vi "Host__MainNewS.vi"() -> ()   [LabVIEW 2018]
uses:
  Master/DAQ/Master_DataControl.ctl
  Master/DAQ/TypeDef_cRIOData.ctl
  Master/IMU/TypeDef_IMUData.ctl
  Master/CAN/TypeDef_BMSData.ctl
  Master/CAN/TypeDef_BMS_Status.ctl
  Master/CAN/MotorController/fixedMotorData.ctl
  Master/CAN/MotorController/MotorStatus.ctl
  Master/Control/TypeDef_DigitalOuts.ctl
  Libraries/TypeDef_CurrentState.ctl
  HealthCheckClass/HealthCheck.lvclass
panel:
  out "Low Side Indicator":bool
  out "Precharge Indicator":bool
  out "Dump Valve":bool
  out "Ignition Indicator":bool
  out "Pump Indicator":bool
  out "High Side Indicator":bool
  out "Clamp Indicator":bool
  out "Brakes Indicator":bool
  out "Pod Power":bool
  out "x Acceleration (g)":dbl(graph)
  out "Speed (mph)":dbl(graph)
  in  "ManualBrake":bool
  in  "ForceIdle":bool
  in  "Pod Power":bool
  out "CurrentState Ind.":u16(ring)
  in  "stop":bool
  in  "Edit Table":bool
  out "HealthCheckTable":string[][](table)
  in  "Tab Control":enum32{"Service", "Systems Check", "Run"}(tab)
  in  "DrvieEnable":bool
  in  "ServiceHOLD":bool
  in  "Service Toggle":bool
  in  "Ignition":bool
  in  "HighSidePermission (SC)":bool caption="High\nSide"
  in  "Brakes (SC)":bool
  in  "Clamp (SC)":bool
  in  "Pump (SC)":bool
  in  "Ignition (SC)":bool
  in  "Low Side (SC)":bool
  in  "Pre-Charge (SC)":bool
  in  "High Side (SC)":bool
  in  "DriveEnable(SC)":bool
  in  "Motor Controller":bool
  in  "Pre-charge":bool
  in  "Ready":bool
  in  "Launch":bool
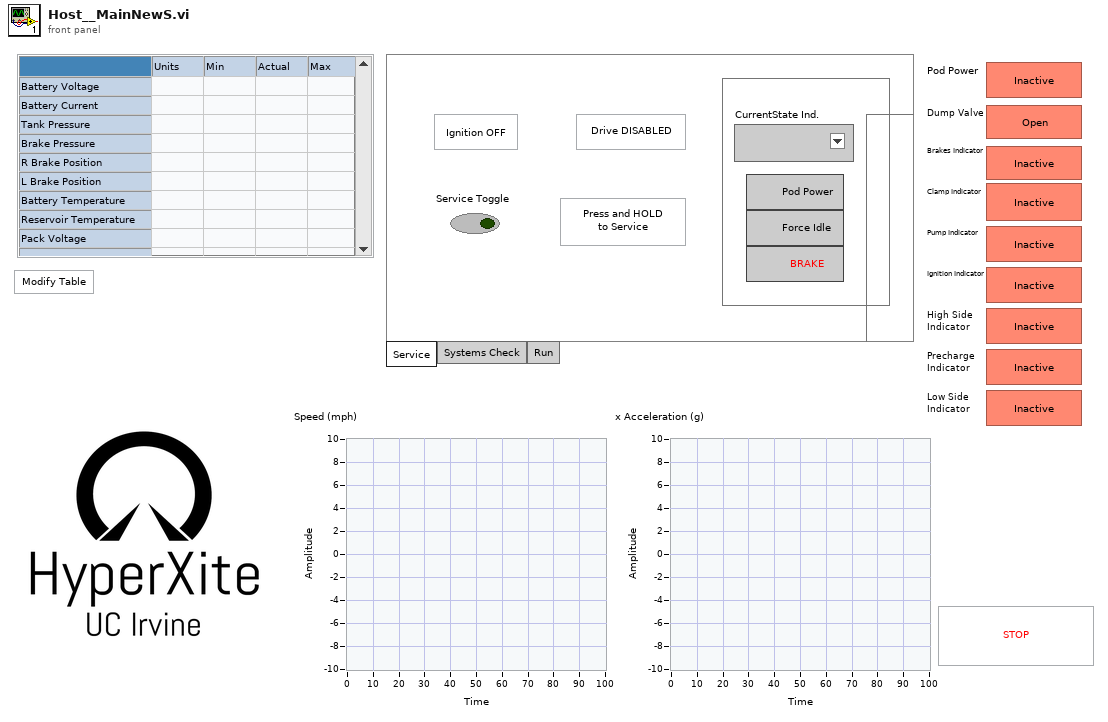
[diagram p1: front panel]
types:
  T1 = enum8{"Enabled", "Disabled", "Disabled and Grayed Out"}
  T2 = typedef "TypeDef_DigitalOuts.ctl" = cluster{"Pod Power":bool, "Dump Valve":bool, "Brakes":bool, "Clamp":bool, "Pump":bool, "Ignition":bool, "DO6":bool, "DO7":bool, "HighSide":bool, "Precharge":bool, "LowSide":bool, "DO3":bool, "DO4":bool, "DO5":bool, "DO62":bool, "DO72":bool}
  T3 = typedef "Master_DataControl.ctl" = cluster{"cRIO Data":T4, "IMU Data":T5, "BMS Data":T6, "Motor Data":T8}
  T4 = typedef "TypeDef_cRIOData.ctl" = cluster{"Time (ms)":dbl, "24V Battery (V)":dbl, "LowV Current (A)":dbl, "Fiducial Sensor (V)":dbl, "PV Pressure (psig)":dbl, "Flow Sensor (V)":dbl, "Temp Fairing (F)":dbl, "Temp Reservoir (F)":dbl, "HallEffect Right (in)":dbl, "HallEffect Left (in)":dbl, "PT Tank (psig)":dbl, "PT Clamp Right (psig)":dbl, "PT Clamp Left (psig)":dbl, "PT Brake (psig)":dbl, "PT Cooling (psig)":dbl, "Displacement (ft)":dbl, "Velocity (ft/s)":dbl}
  T5 = typedef "TypeDef_IMUData.ctl" = cluster{"x acceleration (g)":dbl, "Pressure (psia)":dbl, "Temperature (F)":dbl}
  T6 = typedef "TypeDef_BMSData.ctl" = cluster{"Max Cell Voltage (V)":dbl, "Max Cell ID":dbl, "Min Cell Voltage (V)":dbl, "Min Cell ID":dbl, "State of Charge (%)":dbl, "Average Voltage (V)":dbl, "Voltage Delta (V)":dbl, "Pack Current (A)":dbl, "Pack Voltage (V)":dbl, "Max Resistance (Ohm)":dbl, "Min Resistance (Ohm)":dbl, "Average Resistance (Ohm)":dbl, "Delta Resistance (Ohm)":dbl, "Highest Temperature(F)":dbl, "BmsStatus":T7}
  T7 = typedef "TypeDef_BMS_Status.ctl" = cluster{"isFault":bool, "isolationMonitoring":bool}
  T8 = typedef "fixedMotorData.ctl" = cluster{"Velo (RPM)":dbl, "MotorTemp(F)":dbl, "CtrlTemp(F)":dbl, "DcLinkVolt(V)":dbl, "ErrorCode":dbl, "motorStatus":T9, "isAlive":bool, "motorControllerState":u16}
  T9 = typedef "MotorStatus.ctl" = cluster{"isReady":bool, "isOn":bool, "isOperEn":bool, "isFault":bool, "isVoltEn":bool, "targetReached":bool, "isWarning":bool}
  T10 = typedef "TypeDef_CurrentState.ctl" = enum16{"Fault", "Idle", "Ready", "Pushing", "Coast", "Braking"}
  T11 = typedef "HealthCheck.lvclass/HCState_TypeDef.ctl" = enum16{"Initialization", "Running", "Modify Table"}
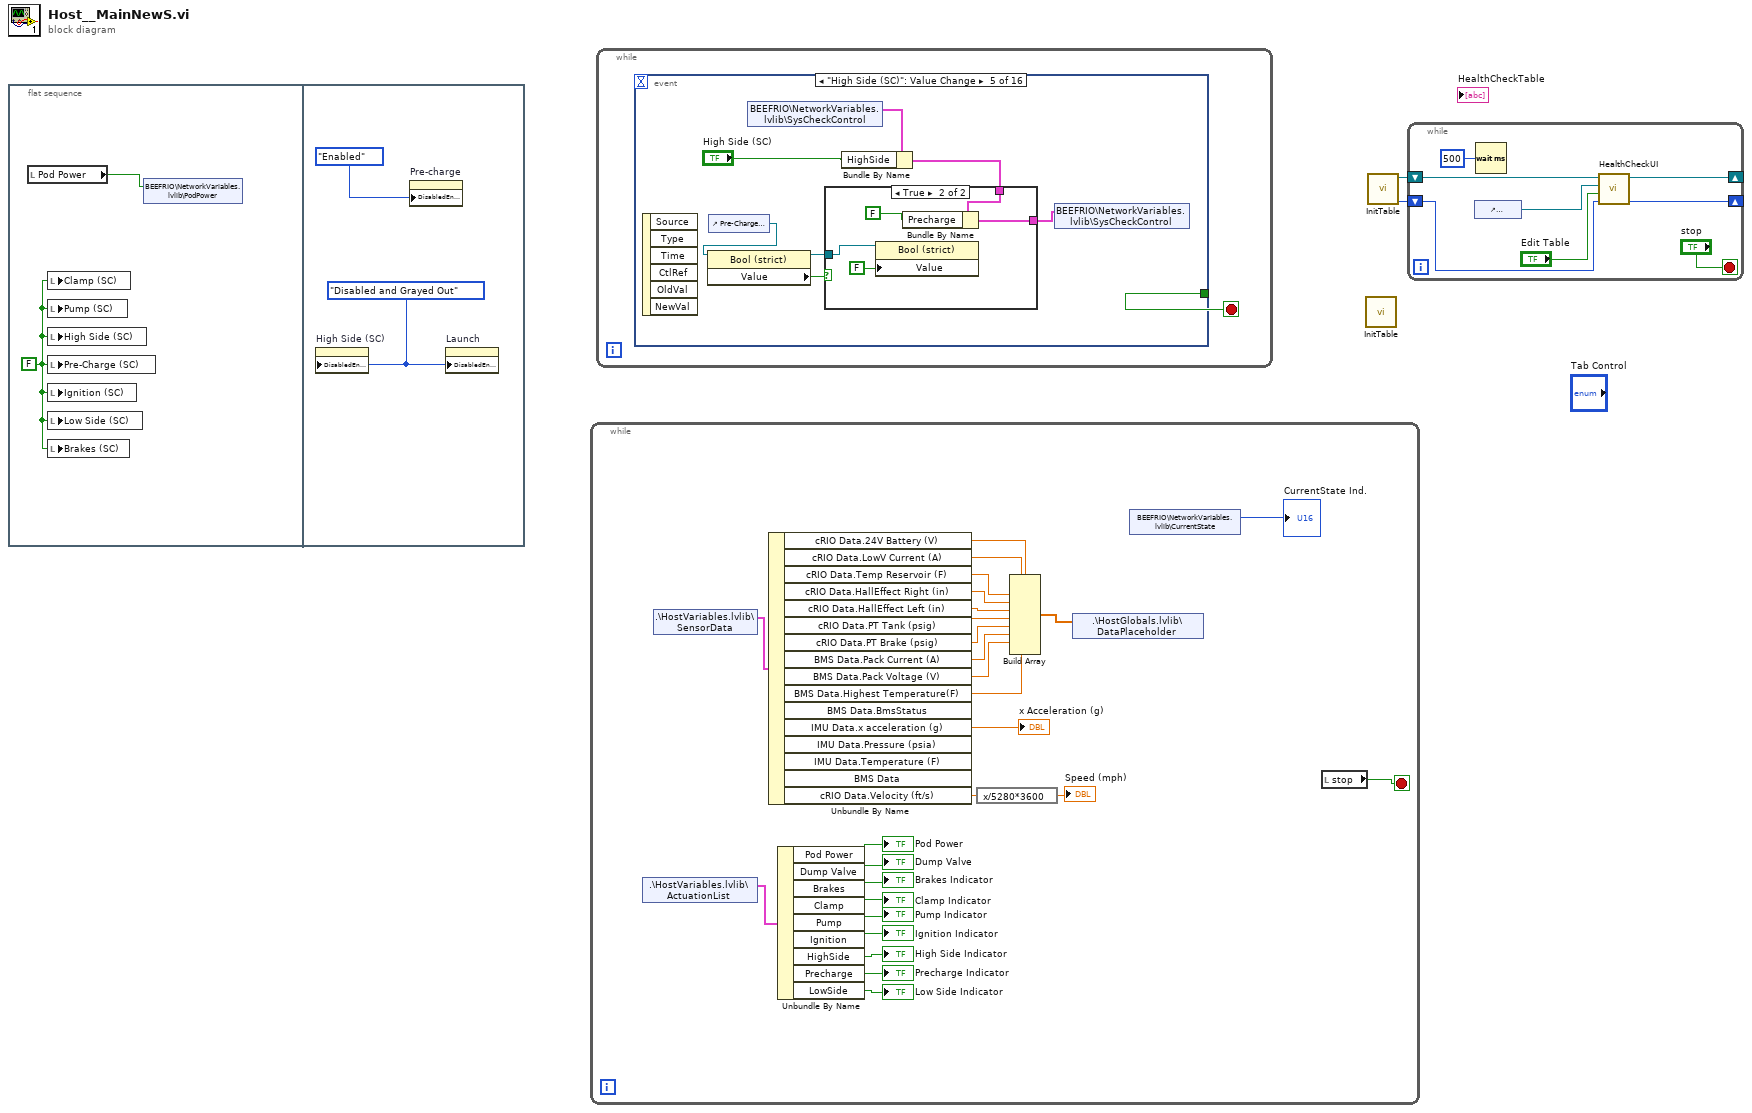
[diagram p0: block diagram]
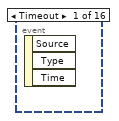
[diagram p2: hidden frame]
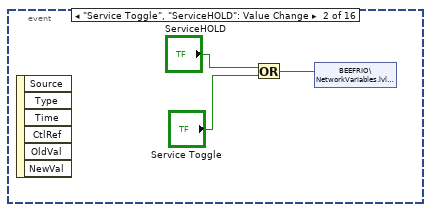
[diagram p3: hidden frame]
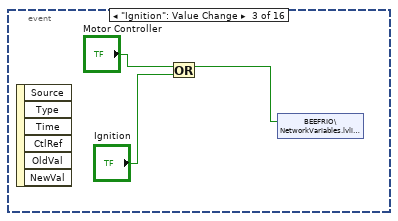
[diagram p4: hidden frame]
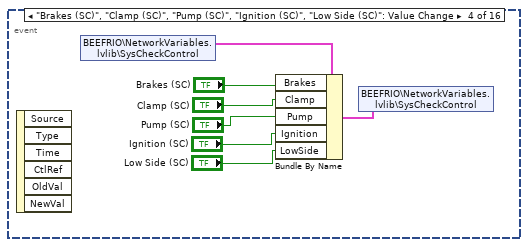
[diagram p5: hidden frame]
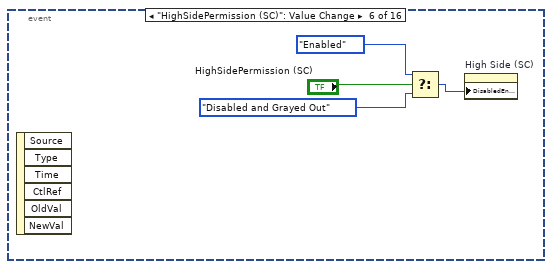
[diagram p7: hidden frame]
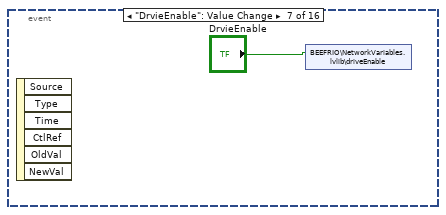
[diagram p8: hidden frame]
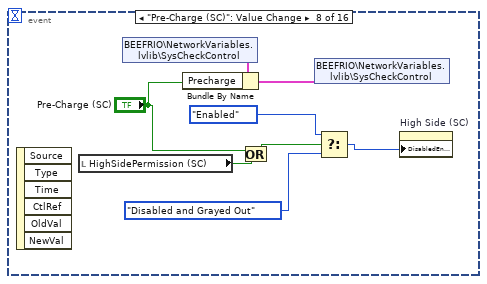
[diagram p9: hidden frame]
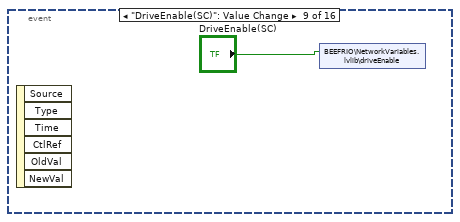
[diagram p10: hidden frame]
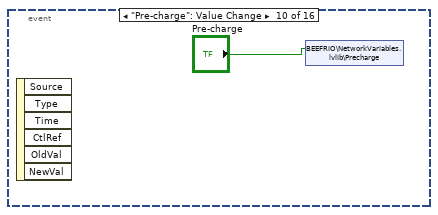
[diagram p11: hidden frame]
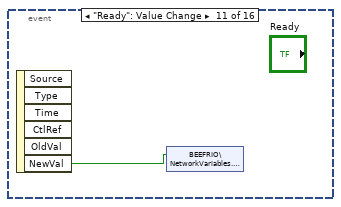
[diagram p12: hidden frame]
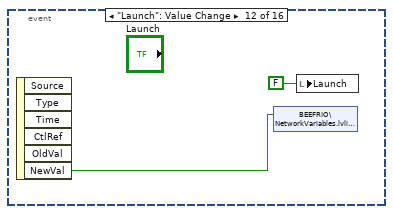
[diagram p13: hidden frame]
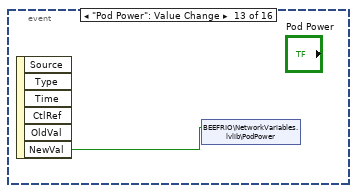
[diagram p14: hidden frame]
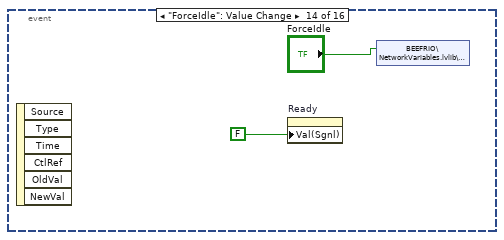
[diagram p15: hidden frame]
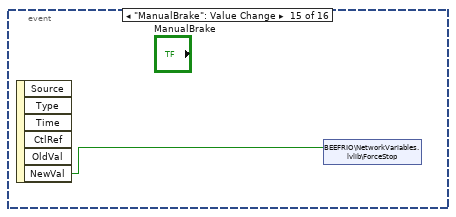
[diagram p16: hidden frame]
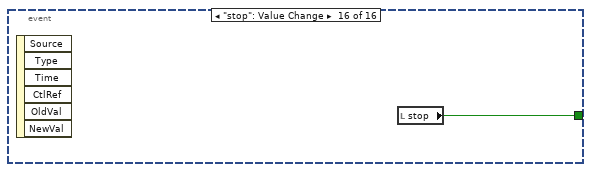
[diagram p17: hidden frame]
diagram:
  n1 = flat-sequence {
    frame #0 {
      w3 = FALSE
      n2 = local read "Pod Power"() -> (w4:bool)
      n3 = local write "Clamp (SC)"(w3) -> ()
      n4 = local write "Pump (SC)"(w3) -> ()
      n5 = local write "High Side (SC)"(w3) -> ()
      n6 = local write "Pre-Charge (SC)"(w3) -> ()
      n7 = local write "Ignition (SC)"(w3) -> ()
      n8 = local write "Low Side (SC)"(w3) -> ()
      n9 = local write "Brakes (SC)"(w3) -> ()
      n10 = shared-variable "BEEFRIO\\NetworkVariables.lvlib\\PodPower"(w4) -> ()  [unwired: 1 in, 1 out]
    }
    frame #1 {
      w5 = T1."Disabled and Grayed Out" ("Disabled")
      n11 = property on="High Side (SC)" class="Bool (strict)"("DisabledEnum"=w5) -> ()  [unwired: 2 in, 2 out]
      n12 = property on="Pre-charge" class="Bool (strict)"("DisabledEnum"=T1."Enabled" ("Disabled")) -> ()  [unwired: 2 in, 2 out]
      n13 = property on="Launch" class="Bool (strict)"("DisabledEnum"=w5) -> ()  [unwired: 2 in, 2 out]
    }
  }
  n14 = while {
    stop <- w21 stop-if-true
    n15 = shared-variable ".\\HostVariables.lvlib\\ActuationList"() -> (w16:T2)  [unwired: 1 in, 1 out]
    n16 = shared-variable ".\\HostVariables.lvlib\\SensorData"() -> (w33:T3)  [unwired: 1 in, 1 out]
    n17 = Unbundle By Name(w33) -> ("cRIO Data.24V Battery (V)"=w32:dbl, "cRIO Data.LowV Current (A)"=w31:dbl, "cRIO Data.Temp Reservoir (F)"=w30:dbl, "cRIO Data.HallEffect Right (in)"=w29:dbl, "cRIO Data.HallEffect Left (in)"=w28:dbl, "cRIO Data.PT Tank (psig)"=w27:dbl, "cRIO Data.PT Brake (psig)"=w26:dbl, "BMS Data.Pack Current (A)"=w25:dbl, "BMS Data.Pack Voltage (V)"=w24:dbl, "BMS Data.Highest Temperature(F)"=w23:dbl, "IMU Data.x acceleration (g)"=→"x Acceleration (g)":dbl, "cRIO Data.Velocity (ft/s)"=w18:dbl)  [unwired: 4 out]
    n18 = Unbundle By Name(w16) -> ("Pod Power"=→"Pod Power":bool, "Dump Valve"=→"Dump Valve":bool, "Brakes"=→"Brakes Indicator":bool, "Clamp"=→"Clamp Indicator":bool, "Pump"=→"Pump Indicator":bool, "Ignition"=→"Ignition Indicator":bool, "HighSide"=→"High Side Indicator":bool, "Precharge"=→"Precharge Indicator":bool, "LowSide"=→"Low Side Indicator":bool)
    n19 = expression code="x/5280*3600"(w18) -> (→"Speed (mph)":dbl)
    n20 = Build Array(w32, w31, w30, w29, w28, w27, w26, w25, w24, w23) -> (w22:dbl[])
    n21 = shared-variable ".\\HostGlobals.lvlib\\DataPlaceholder"(w22) -> ()  [unwired: 1 in, 1 out]
    n22 = shared-variable "BEEFRIO\\NetworkVariables.lvlib\\CurrentState"() -> (→"CurrentState Ind.":T10)  [unwired: 1 in, 1 out]
    n23 = local read "stop"() -> (w21:bool)
  }
  n24 = while {
    stop <- w34 stop-if-true
    n25 = event shown="[4] \"High Side (SC)\": Value Change" {
      selector: _ -> [_ _ _ _ _ _ _ _ _ _ _ _ _ _ _ _]
      dyn-events: _ -> [_ _ _ _ _ _ _ _ _ _ _ _ _ _ _ _]
      timeout: _ -> [_ _ _ _ _ _ _ _ _ _ _ _ _ _ _ _]
      tunnel: [_ _ _ _ _ _ _ _ _ _ _ _ _ _ _ w83] -> w34
      event Timeout {
        n26 = event-data() -> ()  [unwired: 1 in, 3 out]
      }
      event "Service Toggle", "ServiceHOLD": Value Change {
        n27 = event-data() -> ()  [unwired: 1 in, 6 out]
        n28 = Or(x="ServiceHOLD", y="Service Toggle") -> (x .or. y?=w37:bool)
        n29 = shared-variable "BEEFRIO\\NetworkVariables.lvlib\\Service"(w37) -> ()  [unwired: 1 in, 1 out]
      }
      event "Ignition": Value Change {
        n30 = event-data() -> ()  [unwired: 1 in, 6 out]
        n31 = Or(x="Motor Controller", y="Ignition") -> (x .or. y?=w40:bool)
        n32 = shared-variable "BEEFRIO\\NetworkVariables.lvlib\\Ignition"(w40) -> ()  [unwired: 1 in, 1 out]
      }
      event "Brakes (SC)", "Clamp (SC)", "Pump (SC)", "Ignition (SC)", "Low Side (SC)": Value Change {
        n33 = event-data() -> ()  [unwired: 1 in, 6 out]
        n34 = shared-variable "BEEFRIO\\NetworkVariables.lvlib\\SysCheckControl"() -> (w41:T2)  [unwired: 1 in, 1 out]
        n35 = Bundle By Name(cluster=w41, "Brakes"="Brakes (SC)", "Clamp"="Clamp (SC)", "Pump"="Pump (SC)", "Ignition"="Ignition (SC)", "LowSide"="Low Side (SC)") -> (w42:T2)
        n36 = shared-variable "BEEFRIO\\NetworkVariables.lvlib\\SysCheckControl"(w42) -> ()  [unwired: 1 in, 1 out]
      }
      event "High Side (SC)": Value Change {
        n37 = event-data() -> ()  [unwired: 1 in, 6 out]
        n38 = control-ref of="Pre-Charge (SC)"() -> (w53:refnum<vi>)
        n39 = property class="Bool (strict)"(reference=w53) -> (reference out=w52:refnum<vi>, "Value"=w48:bool)  [unwired: 1 in, 1 out]
        n40 = shared-variable "BEEFRIO\\NetworkVariables.lvlib\\SysCheckControl"() -> (w54:T2)  [unwired: 1 in, 1 out]
        n41 = Bundle By Name(cluster=w54, "HighSide"="High Side (SC)") -> (w51:T2)
        n42 = case shown="True" w48 {
          tunnel: w52 -> [_ w59]
          tunnel: w51 -> [w55 w57]
          tunnel: [w55 w56] -> w50
          frame False {
          }
          frame True {
            n43 = property class="Bool (strict)"(reference=w59, "Value"=FALSE) -> ()  [unwired: 1 in, 2 out]
            n44 = Bundle By Name(cluster=w57, "Precharge"=FALSE ("Actuators.PrechargeContactor")) -> (w56:T2)
          }
        }
        n45 = shared-variable "BEEFRIO\\NetworkVariables.lvlib\\SysCheckControl"(w50) -> ()  [unwired: 1 in, 1 out]
      }
      event "HighSidePermission (SC)": Value Change {
        n46 = event-data() -> ()  [unwired: 1 in, 6 out]
        n47 = Select(t=T1."Enabled" ("Disabled"), s="HighSidePermission (SC)", f=T1."Disabled and Grayed Out" ("Disabled")) -> (s? t:f=w61:T1)
        n48 = property on="High Side (SC)" class="Bool (strict)"("DisabledEnum"=w61) -> ()  [unwired: 2 in, 2 out]
      }
      event "DrvieEnable": Value Change {
        n49 = event-data() -> ()  [unwired: 1 in, 6 out]
        n50 = shared-variable "BEEFRIO\\NetworkVariables.lvlib\\driveEnable"("DrvieEnable") -> ()  [unwired: 1 in, 1 out]
      }
      event "Pre-Charge (SC)": Value Change {
        n51 = event-data() -> ()  [unwired: 1 in, 6 out]
        n52 = local read "HighSidePermission (SC)"() -> (w70:bool)
        n53 = shared-variable "BEEFRIO\\NetworkVariables.lvlib\\SysCheckControl"() -> (w73:T2)  [unwired: 1 in, 1 out]
        n54 = Bundle By Name(cluster=w73, "Precharge"="Pre-Charge (SC)") -> (w72:T2)
        n55 = Or(x="Pre-Charge (SC)", y=w70) -> (x .or. y?=w71:bool)
        n56 = shared-variable "BEEFRIO\\NetworkVariables.lvlib\\SysCheckControl"(w72) -> ()  [unwired: 1 in, 1 out]
        n57 = Select(t=T1."Enabled" ("Disabled"), s=w71, f=T1."Disabled and Grayed Out" ("Disabled")) -> (s? t:f=w67:T1)
        n58 = property on="High Side (SC)" class="Bool (strict)"("DisabledEnum"=w67) -> ()  [unwired: 2 in, 2 out]
      }
      event "DriveEnable(SC)": Value Change {
        n59 = event-data() -> ()  [unwired: 1 in, 6 out]
        n60 = shared-variable "BEEFRIO\\NetworkVariables.lvlib\\driveEnable"("DriveEnable(SC)") -> ()  [unwired: 1 in, 1 out]
      }
      event "Pre-charge": Value Change {
        n61 = event-data() -> ()  [unwired: 1 in, 6 out]
        n62 = shared-variable "BEEFRIO\\NetworkVariables.lvlib\\Precharge"("Pre-charge") -> ()  [unwired: 1 in, 1 out]
      }
      event "Ready": Value Change {
        n63 = event-data() -> ("NewVal"=w76:bool)  [unwired: 1 in, 5 out]
        n64 = shared-variable "BEEFRIO\\NetworkVariables.lvlib\\Ready"(w76) -> ()  [unwired: 1 in, 1 out]
      }
      event "Launch": Value Change {
        n65 = event-data() -> ("NewVal"=w77:bool)  [unwired: 1 in, 5 out]
        n66 = shared-variable "BEEFRIO\\NetworkVariables.lvlib\\Launch"(w77) -> ()  [unwired: 1 in, 1 out]
        n67 = local write "Launch"(FALSE ("Ready")) -> ()
      }
      event "Pod Power": Value Change {
        n68 = event-data() -> ("NewVal"=w79:bool)  [unwired: 1 in, 5 out]
        n69 = shared-variable "BEEFRIO\\NetworkVariables.lvlib\\PodPower"(w79) -> ()  [unwired: 1 in, 1 out]
      }
      event "ForceIdle": Value Change {
        n70 = event-data() -> ()  [unwired: 1 in, 6 out]
        n71 = property on="Ready" class="Bool (strict)"("Val(Sgnl)"=FALSE) -> ()  [unwired: 2 in, 2 out]
        n72 = shared-variable "BEEFRIO\\NetworkVariables.lvlib\\ForceIdle"("ForceIdle") -> ()  [unwired: 1 in, 1 out]
      }
      event "ManualBrake": Value Change {
        n73 = event-data() -> ("NewVal"=w82:bool)  [unwired: 1 in, 5 out]
        n74 = shared-variable "BEEFRIO\\NetworkVariables.lvlib\\ForceStop"(w82) -> ()  [unwired: 1 in, 1 out]
      }
      event "stop": Value Change {
        n75 = event-data() -> ()  [unwired: 1 in, 6 out]
        n76 = local read "stop"() -> (w83:bool)
      }
    }
  }
  n77 = call "InitTable.vi"() -> ()  [unwired: 10 in, 2 out]
  n78 = call "InitTable.vi"() -> ("Enum out"=w1:T11, "HealthCheck out"=w2:refnum<class "HealthCheck.lvclass">)  [unwired: 10 in]
  n79 = while {
    shift-right: [w87] -> _
    shift-left: w2 -> [w86]
    shift-right: [w85] -> _
    shift-left: w1 -> [w84]
    stop <- "stop" stop-if-true
    n80 = control-ref of="HealthCheckTable"() -> (w88:refnum<vi>)
    n81 = Wait (ms)(milliseconds to wait=u32 500) -> ()  [unwired: 1 out]
    n82 = call "HealthCheckUI.vi"("Enum in"=w84, "Edit Table"="Edit Table", "Table in"=w88, "HealthCheck.lvclass"=w86) -> ("Enum out"=w85:T11, "HealthCheck out"=w87:refnum<class "HealthCheck.lvclass">)  [unwired: 6 in]
  }
